vi "Build.vi"(9 "long name":string, 10 "file name":string, 11 "file attributes":T1 {"permissions" format="%04o"}) -> (3 "file attributes out":refnum<class "File Attributes.lvclass">)   [LabVIEW 2020, in "NI_SFTP.lvlib" / "File Attributes.lvclass"]
uses:
  <vilib>/net/SFTP/File Attributes/File Attributes.lvclass
  <vilib>/net/SFTP/API/Support/File Attributes.ctl
  <vilib>/net/SFTP/File Attributes/File Attributes.lvclass/File Attributes.ctl
  <vilib>/net/SFTP/NI_SFTP.lvlib
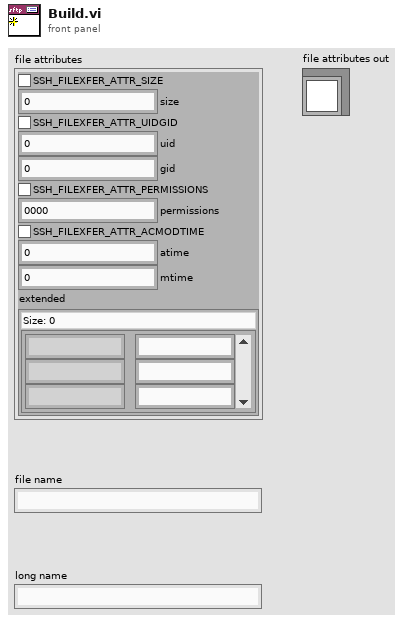
[diagram p1: front panel]
types:
  T1 = typedef "NI_SFTP.lvlib/File Attributes.ctl" = cluster{"SSH_FILEXFER_ATTR_SIZE":bool, "size":u64, "SSH_FILEXFER_ATTR_UIDGID":bool, "uid":u32, "gid":u32, "SSH_FILEXFER_ATTR_PERMISSIONS":bool, "permissions":u32, "SSH_FILEXFER_ATTR_ACMODTIME":bool, "atime":u32, "mtime":u32, "extended":map{string, string}}
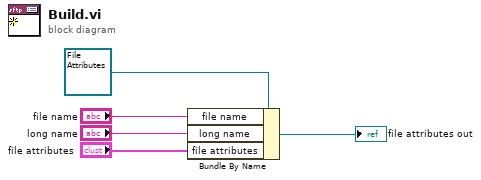
[diagram p0: block diagram]
diagram:
  n1 = Bundle By Name(cluster=refnum<class "File Attributes.lvclass"> refnum ("SFTP File Attributes in"), "file name"="file name", "long name"="long name", "file attributes"="file attributes") -> (→"file attributes out":refnum<class "File Attributes.lvclass">)
